vi "拉压力传感器参数.vi"(8 "写入数据":u32, 9 "写入地址":u32=22, 10 "枚举":enum16{"读取", "写入"}(ring)) -> (3 "拉压测试状态":dbl format="%#_8g")   [LabVIEW 2019]
uses:
  S7/S7Ref.vi
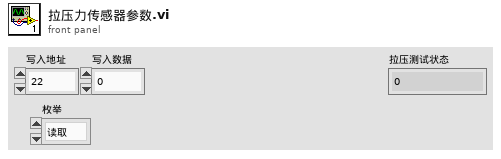
[diagram p1: front panel]
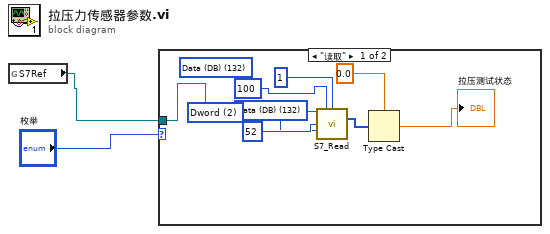
[diagram p0: block diagram]
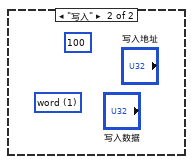
[diagram p2: hidden frame]
diagram:
  n1 = global read "S7Ref.vi" "S7Ref"() -> (w1:refnum<k5>)
  n2 = case shown="\"读取\"" "枚举" {
    tunnel: w1 -> [w6 _]
    frame "读取" {
      w3 = u8 132 items=["I/O (P)"=128, "Input (I)"=129, "Output (Q)"=130, "Bit Memory (M)"=131, "Data (DB)"=132, "Instance Data (DI)"=133, "Local Data (L)"=134, "Predecessor Local Data (VL)"=135] ("寄存器类型")
      (unwired) u8 132 items=["I/O (P)"=128, "Input (I)"=129, "Output (Q)"=130, "Bit Memory (M)"=131, "Data (DB)"=132, "Instance Data (DI)"=133, "Local Data (L)"=134, "Predecessor Local Data (VL)"=135] ("寄存器类型")
      w4 = u16 2 items=["byte", "word", "Dword"] ("数据类型")
      n3 = call "S7_Read.vi"("TCP"=w6, "DB #"=u16 100, "读取长度"=u16 1, "寄存器类型"=w3, "起始地址"=u32 52, "数据类型"=w4) -> ("数据"=w9:u32[])  [unwired: 6 in, 3 out]
      n4 = Type Cast(type=0.0, x=w9) -> (*(type *) &x=→"拉压测试状态":dbl)
    }
    frame "写入" {
      (unwired) u16 1 items=["byte", "word", "Dword"] ("数据类型")
      (unwired) u16 100 ("DB #")
    }
  }
